vi "niScope Cal Set Accessory Source.vi"(8 "error in":errorcluster {"code" format="%.0x"}, 9 "calSource":i32(ring) items=["+10V"=1, "GND"=0, "-10V"=2], 10 "channels":string="0", 11 "instrument handle":refnum<k15>) -> (0 "error out":errorcluster={"status"=FALSE, "code"=0, "source"="\n\n"} {"code" format="%.0x"}, 3 "instrument handle out":refnum<k15>)   [LabVIEW 2011]
doc: "For the NI 5900 differential amplifier, this VI connects the specified channel to the calibration source and sets the calibration source to +/-10 V or to GND."
uses:
  niScope_32.dll
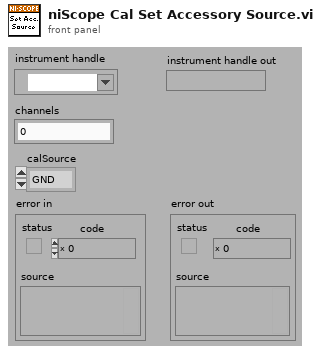
[diagram p1: front panel]
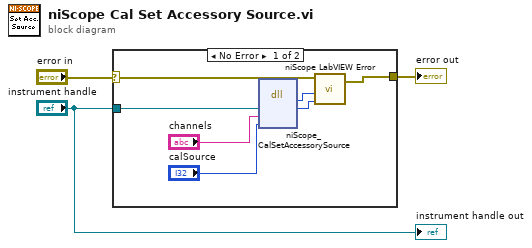
[diagram p0: block diagram]
diagram:
  n1 = case shown="No Error" "error in" {
    selector: "error in" -> [w10 w11]
    tunnel: [w9 w11] -> w2
    tunnel: "instrument handle" -> [w6 _]
    frame No Error {
      n2 = dll-call lib="niScope_*.*" fn="niScope_CalSetAccessorySource"("instrumentHandle"=w6, "channelName"="channels", "calSource"="calSource") -> (w8:i32, "instrumentHandle"=w7:i32)  [unwired: 5 in, 2 out]
      n3 = call <instrlib>:"niScope LabVIEW Error.vi"("instrument handle"=w7, "niScope error code (0)"=w8, "error in (no error)"=w10) -> ("error out"=w9:errorcluster)  [unwired: 2 in]
    }
    frame Error {
    }
  }
  "error out" <- w2
  "instrument handle out" <- "instrument handle"
